vi "Serialize.vi"(8 "error in (no error)":errorcluster, 11 "RandomNumberLogger Controller in":refnum<class "RandomNumberLogger Controller.lvclass">) -> (0 "error out":errorcluster, 2 "Serialized PE Specification":string, 3 "RandomNumberLogger Controller out":refnum<class "RandomNumberLogger Controller.lvclass">)   [LabVIEW 2020, in "RandomNumberLogger.lvlib" / "RandomNumberLogger Controller.lvclass"]
doc: "<b>Serialize</b>\nProvides the seralized configuration data stored in the plugin controller's class data."
uses:
  RandomNumberLogger Controller.lvclass
  RandomNumberLogger Controller.lvclass/RandomNumberLogger Controller.ctl
  PE/Get Configuration Version.vi
  <vilib>/ADAS Record/Utilities/Config/Data Converter/Data Container and Version to JSON.vi
  PE/RandomNumberLogger.lvclass
panel:
  # "#via_ignore"
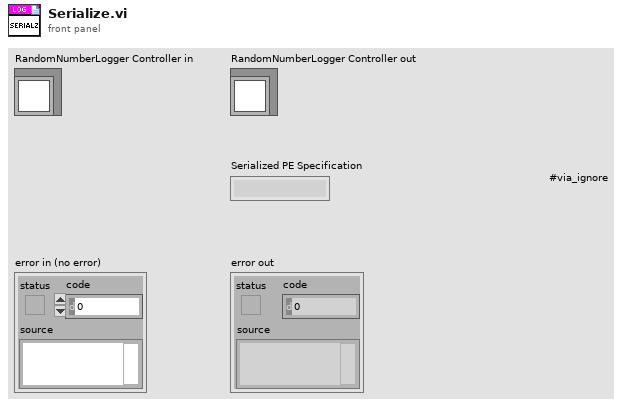
[diagram p1: front panel]
types:
  T1 = typedef "RandomNumberLogger.lvlib/RandomNumberLogger.lvclass/Configuration.ctl" = cluster{"Parameter1":string}
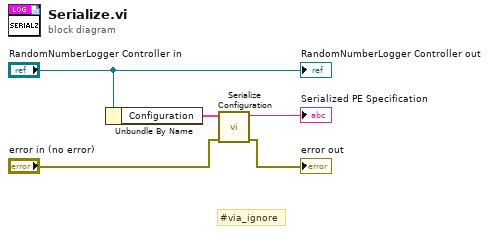
[diagram p0: block diagram]
diagram:
  # "#via_ignore"
  n1 = Unbundle By Name("RandomNumberLogger Controller in") -> ("Configuration"=w4:T1)
  n2 = call "Serialize Configuration.vi"("error in (no error)"="error in (no error)", "Configuration"=w4) -> ("error out"=→"error out":errorcluster, "Serialized Configuration"=→"Serialized PE Specification":string)  [unwired: 8 in]
  "RandomNumberLogger Controller out" <- "RandomNumberLogger Controller in"
